vi "ReadExampleFiles.vi"(11 "Folder":path) -> ()   [LabVIEW 2020]
uses:
  ColorText/Code.xctl
panel:
  in  "Done":bool
  out "Code":string(xcontrol)="import os\n\nfor i in range(10):\n     print(i)\n"
  in  "Files":i32(listbox)
  in  "Folder":u16(ring) items=["Examples"]
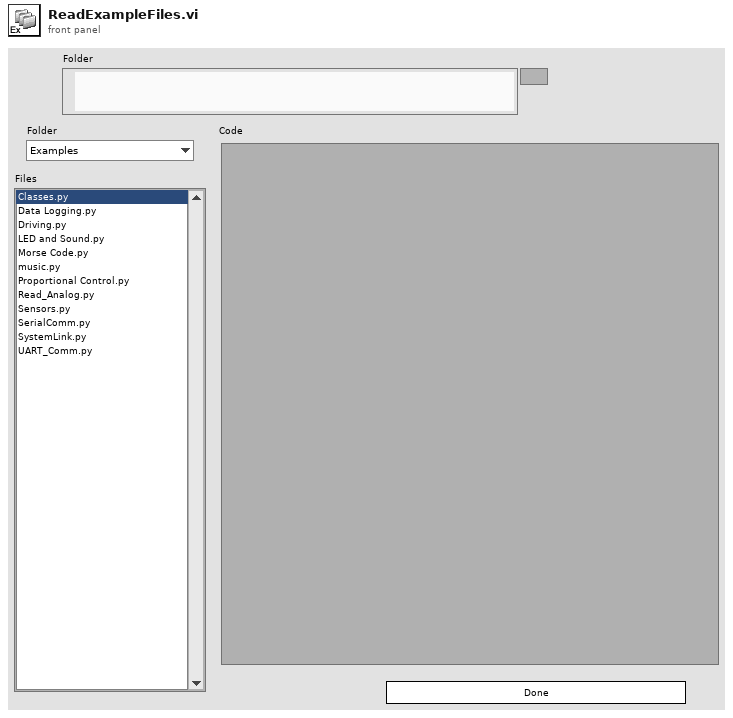
[diagram p1: front panel]
types:
  T1 = enum32{"Invalid", "Standard", "Closed", "Hidden", "Minimized", "Maximized"}
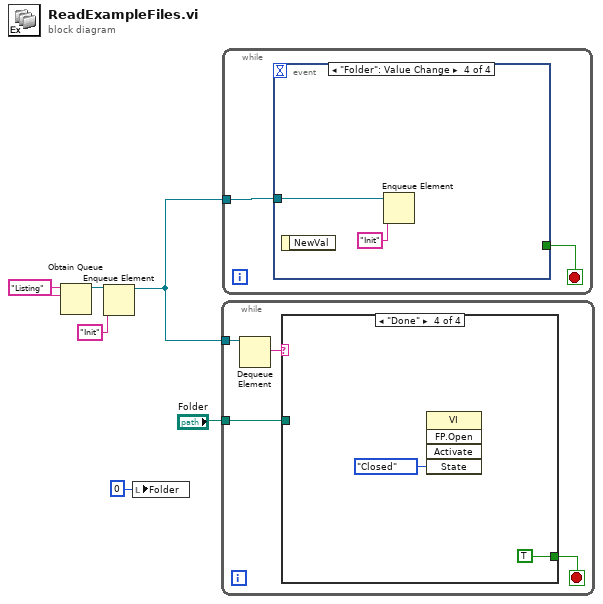
[diagram p0: block diagram]
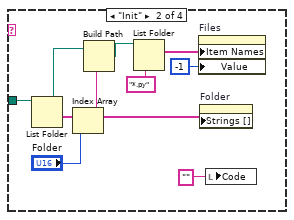
[diagram p3: hidden frame]
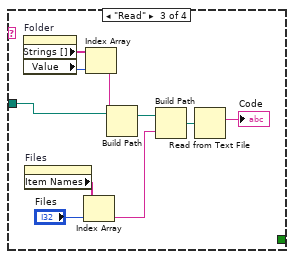
[diagram p4: hidden frame]
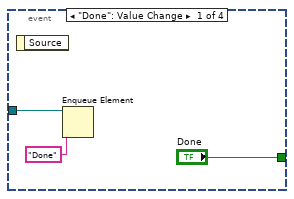
[diagram p5: hidden frame]
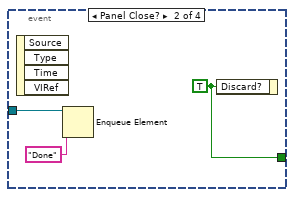
[diagram p6: hidden frame]
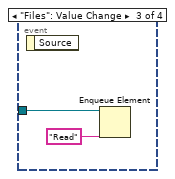
[diagram p7: hidden frame]
diagram:
  w5 = "Listing" ("name (unnamed)")
  n1 = Obtain Queue(name (unnamed)=w5, element data type=w5) -> (queue out=w6:refnum<queue>)  [unwired: 3 in, 2 out]
  n2 = Enqueue Element(queue=w6, element="Init") -> (queue out=w3:refnum<queue>)  [unwired: 2 in, 2 out]
  n3 = local write "Folder"(0 ("Files")) -> ()
  n4 = while {
    tunnel: w3 -> [w10]
    tunnel: "Folder" -> [w7]
    stop <- w8 stop-if-true
    n5 = Dequeue Element(queue=w10) -> (element=w9:string)  [unwired: 2 in, 3 out]
    n6 = case shown="\"Done\"" w9 {
      tunnel: [_ _ _ TRUE] -> w8
      tunnel: w7 -> [_ w13 w22 _]
      frame Default {
      }
      frame "Init" {
        n7 = List Folder(path=w13) -> (folder names=w15:string[])  [unwired: 3 in, 3 out]
        n8 = Index Array(array=w15, index="Folder") -> (element=w14:string)
        n9 = Build Path(base path=w13, name or relative path=w14) -> (appended path=w12:path)
        n10 = List Folder(path=w12, pattern="*.py") -> (filenames=w17:string[])  [unwired: 2 in, 3 out]
        n11 = property on="Files" class="LstBox (strict)"("Item Names"=w17, "Value"=-1 ("Files")) -> ()  [unwired: 2 in, 2 out]
        n12 = property on="Folder" class="Ring (strict)"("Strings []"=w15) -> ()  [unwired: 2 in, 2 out]
        n13 = local write "Code"("") -> ()
      }
      frame "Read" {
        n14 = property on="Folder" class="Ring (strict)"() -> ("Strings []"=w24:string[], "Value"=w23:u16)  [unwired: 2 in, 2 out]
        n15 = property on="Files" class="LstBox (strict)"() -> ("Item Names"=w29:string[])  [unwired: 2 in, 2 out]
        n16 = Index Array(array=w29, index="Files") -> (element=w27:string)
        n17 = Index Array(array=w24, index=w23) -> (element=w20:string)
        n18 = Build Path(base path=w22, name or relative path=w20) -> (appended path=w21:path)
        n19 = Build Path(base path=w21, name or relative path=w27) -> (appended path=w26:path)
        n20 = Read from Text File(file (use dialog)=w26) -> (text=→"Code":string)  [unwired: 3 in, 3 out]
      }
      frame "Done" {
        n21 = invoke class="VI" method="FP.Open"("State"=T1."Closed") -> ()  [unwired: 4 in, 5 out]
      }
    }
  }
  n22 = while {
    tunnel: w3 -> [w32]
    stop <- w33 stop-if-true
    n23 = event shown="[3] \"Folder\": Value Change" {
      selector: _ -> [_ _ _ _]
      dyn-events: _ -> [_ _ _ _]
      timeout: _ -> [_ _ _ _]
      tunnel: ["Done" w37 _ _] -> w33
      tunnel: w32 -> [w34 w38 w40 w42]
      event "Done": Value Change {
        n24 = event-data() -> ()  [unwired: 1 in, 1 out]
        n25 = Enqueue Element(queue=w34, element="Done") -> ()  [unwired: 2 in, 3 out]
      }
      event Panel Close? {
        w37 = TRUE ("Discard?")
        n26 = event-data() -> ()  [unwired: 1 in, 4 out]
        n27 = Enqueue Element(queue=w38, element="Done") -> ()  [unwired: 2 in, 3 out]
        n28 = event-data("Discard?"=w37) -> ()  [unwired: 1 in, 1 out]
      }
      event "Files": Value Change {
        n29 = event-data() -> ()  [unwired: 1 in, 1 out]
        n30 = Enqueue Element(queue=w40, element="Read") -> ()  [unwired: 2 in, 3 out]
      }
      event "Folder": Value Change {
        n31 = event-data() -> ()  [unwired: 1 in, 1 out]
        n32 = Enqueue Element(queue=w42, element="Init") -> ()  [unwired: 2 in, 3 out]
      }
    }
  }
